vi "save.volumes.vi"(8 "error in (no error)":errorcluster, 10 "volume ids":i32[](array[numeric]), 11 "manager_daemon in":refnum<class "manager_daemon.lvclass">) -> (0 "error out":errorcluster, 3 "manager_daemon out":refnum<class "manager_daemon.lvclass">)   [LabVIEW 2024, in "manager_daemon.lvclass"]
uses:
  manager_daemon.lvclass
  manager_daemon.lvclass/manager_daemon.ctl
  CV_Shared_Library/volume.type--enum.ctl
  CV_Shared_Library/CV_Shared_Library.lvlib
  CV_RESTful_Library/typedefs/local_volume--cluster.ctl
  CV_RESTful_Library/CV_RESTful_Lib.lvlib
  <vilib>/addons/_JKI.lib/Serialization/JSON/JKI JSON Serialization.lvlib
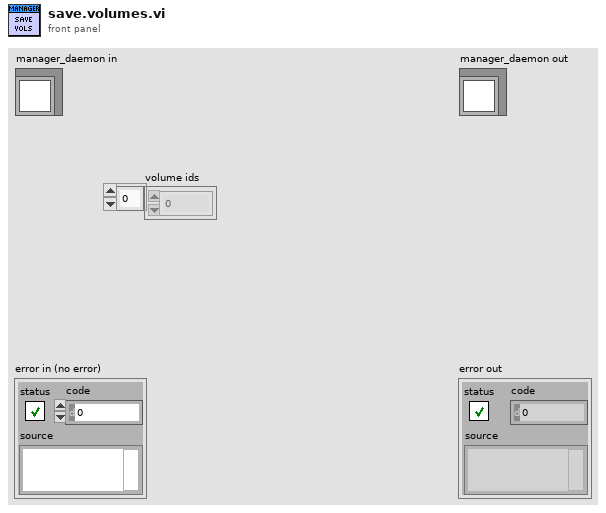
[diagram p1: front panel]
types:
  T1 = typedef "manager_daemon.lvclass/VolumeData--cluster.ctl" = cluster{"name":string, "sortable_name":string, "aliases":string[], "description":string, "site_detail_url":string, "count_of_issues":i32, "start_year":i32, "publisher_id":i32, "issue_ids":i32[], "date_last_updated":timestamp, "volume":i32, "cv_id":string, "volume type":T2, "source_path":path}
  T2 = typedef "CV_Shared_Library.lvlib/volume.type--enum.ctl" = enum16{"Ongoing", "Limited Series", "Annual", "One Shot", "Reprint/Document", "Digital"}
  T3 = typedef "CV_RESTful_Lib.lvlib/local_volume--cluster.ctl" = cluster{"id":i32, "name":string, "sortable_name":string, "aliases":string[], "description":string, "site_detail_url":string, "count_of_issues":i32, "start_year":i32, "publisher_id":i32, "issue_ids":i32[], "date_last_updated":timestamp, "volume":i32, "cv_id":string, "volume type":T2}
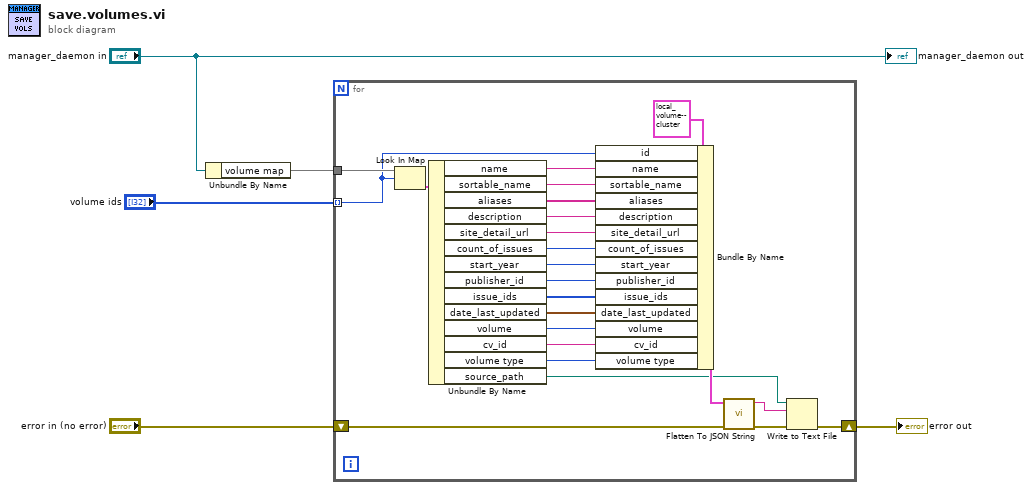
[diagram p0: block diagram]
diagram:
  n1 = Unbundle By Name("manager_daemon in") -> ("volume map"=w5:map{i32, T1})
  n2 = for {
    tunnel: w5 -> [w28]
    tunnel: "volume ids" -> [w26] mode=indexing
    shift-right: [w6] -> w1
    shift-left: "error in (no error)" -> [w7]
    n3 = Look In Map(map=w28, key=w26) -> (value=w25:T1)  [unwired: 1 in, 1 out]
    n4 = Unbundle By Name(w25) -> ("name"=w24:string, "sortable_name"=w23:string, "aliases"=w22:string[], "description"=w21:string, "site_detail_url"=w20:string, "count_of_issues"=w19:i32, "start_year"=w18:i32, "publisher_id"=w17:i32, "issue_ids"=w16:i32[], "date_last_updated"=w15:timestamp, "volume"=w14:i32, "cv_id"=w13:string, "volume type"=w12:T2, "source_path"=w8:path)
    n5 = Bundle By Name(cluster=T3 {"id"=149574, "name"="Mighty Marvel Masterworks: Captain America", "sortable_name"="mighty marvel masterworks- captain america (2022)", "aliases"=[], "description"="<p>A series of Trade Paperbacks collecting material from <a href=\"/tales-of-suspense/4050-2007/\" data-ref-id=\"4050-2007\">Tales of Suspense</a> (1959) </p><ul><li>Volume 1: <span>Collects material from Tales Of Suspense (1959) #59-77</span></li><li><span><span><span>Volume 2: Collects material from TALES OF SUSPENSE (1959) #78-94 and NOT BRAND ECHH #3<br /></span></span></span></li></ul>", "site_detail_url"="https://comicvine.gamespot.com/mighty-marvel-masterworks-captain-america/4050-149574/", "count_of_issues"=3, "start_year"=2022, "publisher_id"=31, "issue_ids"=[984348, 996023, 1047297], "date_last_updated"=timestamp(3781611525 s since 1904-01-01), "volume"=0, "cv_id"="4050-149574", "volume type"=enum."One Shot"} ("volume"), "id"=w26, "name"=w24, "sortable_name"=w23, "aliases"=w22, "description"=w21, "site_detail_url"=w20, "count_of_issues"=w19, "start_year"=w18, "publisher_id"=w17, "issue_ids"=w16, "date_last_updated"=w15, "volume"=w14, "cv_id"=w13, "volume type"=w12) -> (w11:T3)
    n6 = call <vilib>:"Flatten To JSON String.vi"("error in"=w7, "Variant"=w11) -> ("error out"=w9:errorcluster, "JSON String"=w10:string)  [unwired: 8 in]
    n7 = Write to Text File(file (use dialog)=w8, text=w10, error in=w9) -> (error out=w6:errorcluster)  [unwired: 1 in, 2 out]
  }
  "error out" <- w1
  "manager_daemon out" <- "manager_daemon in"
